vi "Vision_Test.vi"() -> ()   [LabVIEW 2017]
uses:
  <vilib>/NI_Real-Time Target Support.lvlib
panel:
  out "Iteration":i32
  out "CPU Load":dbl(graph)
  in  "stop":bool
  out "Image Out":T1(plugin-control)
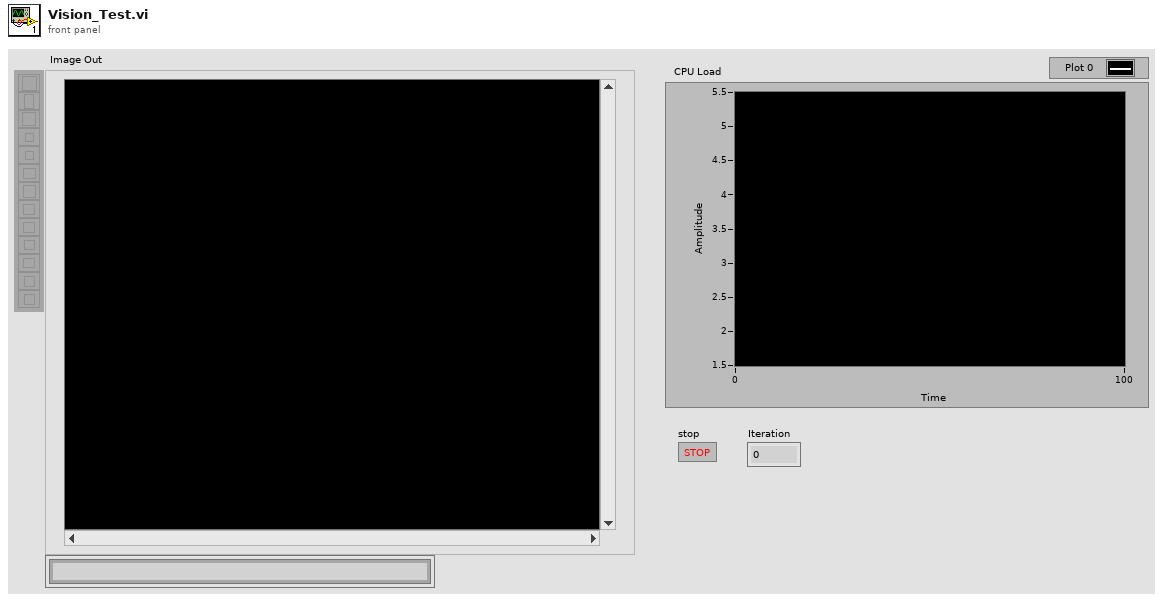
[diagram p1: front panel]
types:
  T1 = typedef "IMAQ Image.ctl" = refnum<image>
  T2 = typedef "NI_Real-Time Target Support.lvlib/RT CPU Load.ctl" = cluster{"Total (%)":dbl, "Time Critical (%)":dbl, "Timed Structures (%)":dbl, "High (%)":dbl, "Above Normal (%)":dbl, "Normal (%)":dbl, "Background (%)":dbl, "Idle (%)":dbl, "ISR (%)":dbl}
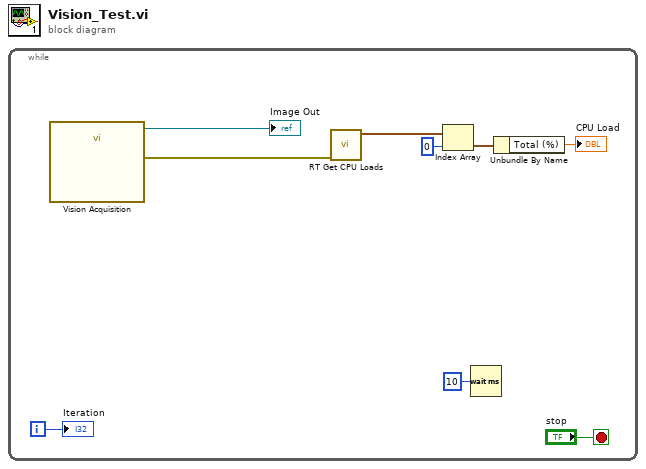
[diagram p0: block diagram]
diagram:
  n1 = while {
    i -> [w2]
    stop <- "stop" stop-if-true
    n2 = call "Vision Acquisition"() -> ("Image Out"=→"Image Out":T1, "error out"=w8:errorcluster)  [unwired: 26 in]
    n3 = call <vilib>:"RT Get CPU Loads.vi"("error in (no error)"=w8) -> ("CPU loads"=w7:T2[])  [unwired: 9 in, 1 out]
    n4 = Index Array(array=w7, index=0) -> (element=w5:T2)
    n5 = Wait (ms)(milliseconds to wait=u32 10) -> ()  [unwired: 1 out]
    n6 = Unbundle By Name(w5) -> ("Total (%)"=→"CPU Load":dbl)
    "Iteration" <- w2
  }
